vi "subGetItemInfosFromProjectFile.vi"(11 "All Files in Dir":path[](array[path])) -> (1 "Source dist":map{string, set{string}}(c390), 2 "TargetFile name":set{string}(c389), 3 "TargetFile info":T1)   [LabVIEW 2020, in "SolutionBuilder.lvlib"]
uses:
  SolutionBuilder.lvlib
  ItemInfo.ctl
  ProjectInfo.ctl
  FileInfo.ctl
  <vilib>/xml/Load XML File.vi
  <vilib>/xml/Close Reference(Node).vi
  <vilib>/xml/NI_XML.lvlib
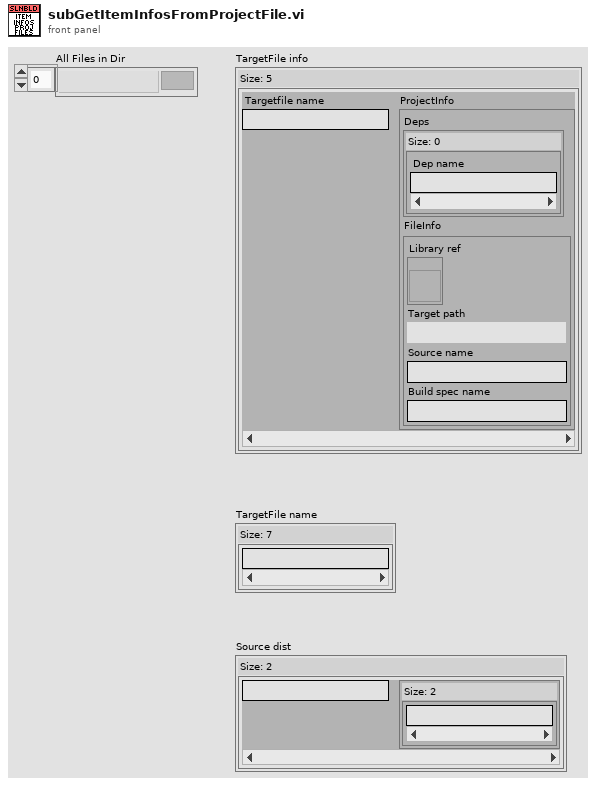
[diagram p1: front panel]
types:
  T1 = typedef "SolutionBuilder.lvlib/ItemInfo.ctl" = map{string, T2}
  T2 = typedef "SolutionBuilder.lvlib/ProjectInfo.ctl" = cluster{"Deps":set{string}, "FileInfo":T3}
  T3 = typedef "SolutionBuilder.lvlib/FileInfo.ctl" = cluster{"Library ref":refnum<vi>, "Target path":path, "Source name":string, "Build spec name":string}
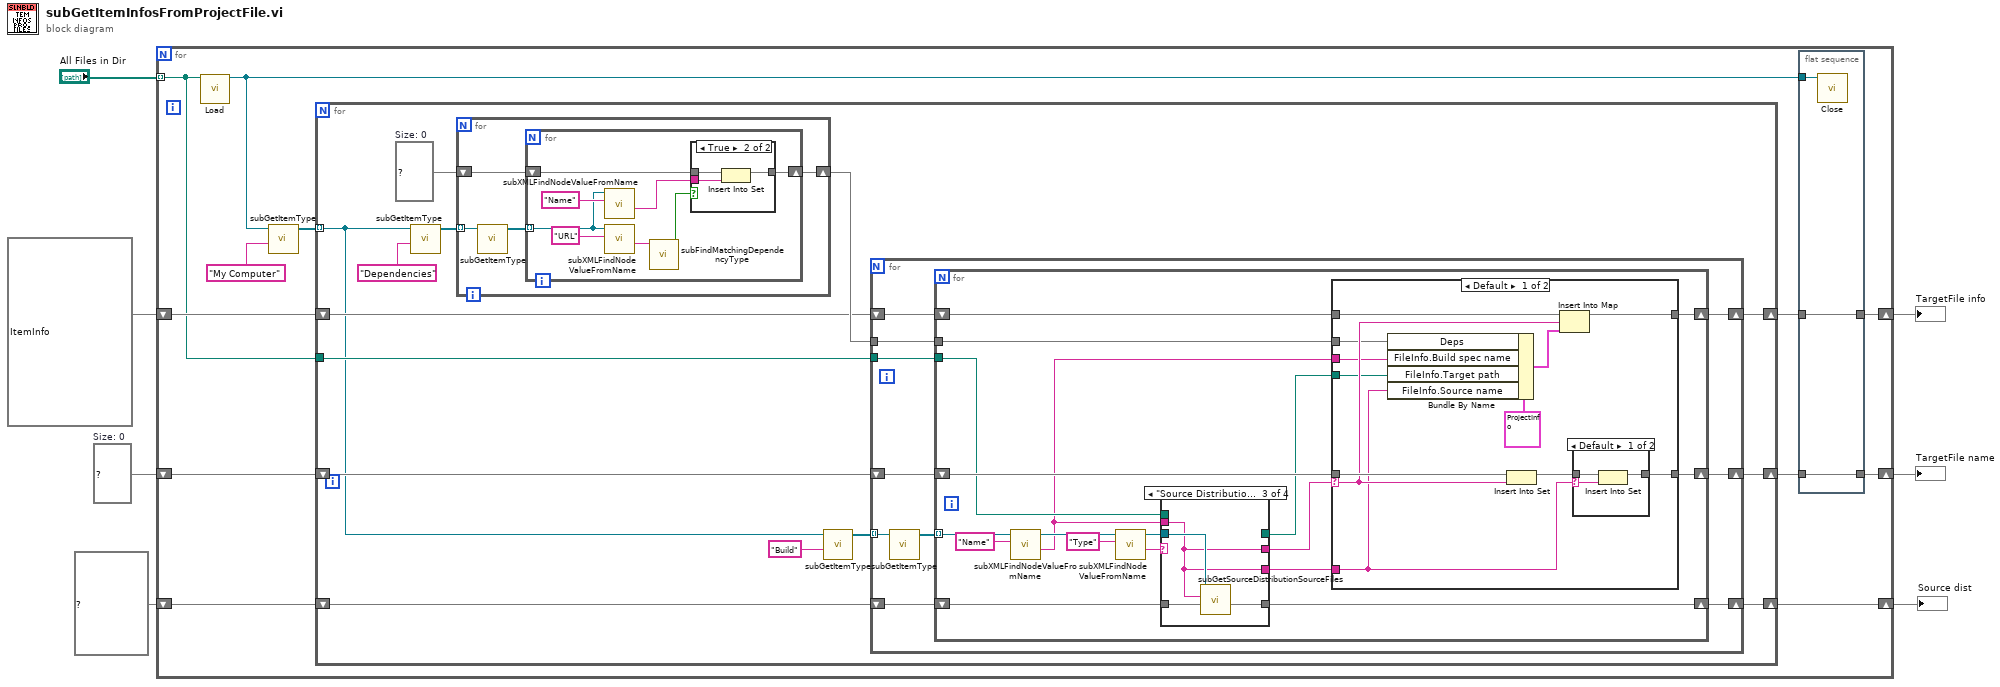
[diagram p0: block diagram]
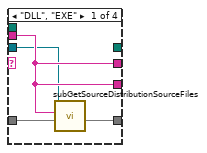
[diagram p3: hidden frame]
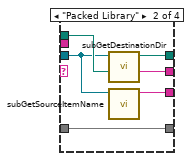
[diagram p4: hidden frame]
diagram:
  w4 = set{string} {}  # Size: 0
  n1 = for {
    tunnel: "All Files in Dir" -> [w10] mode=indexing
    shift-right: [w12] -> w5
    shift-left: w4 -> [w14]
    shift-right: [w13] -> w6
    shift-left: T1 {} ("map in") -> [w15]
    shift-right: [w9] -> w1
    shift-left: map{string, set{string}} {} ("Source dist") -> [w8]
    n2 = call-poly <vilib>:"Load.vi"("path to XML document"=w10) -> ("DOM document out"=w11:refnum<k20>)  [unwired: 12 in, 2 out]
    n3 = call "subGetItemType.vi"("Property value"="My Computer", "Refnum in"=w11) -> ("Nodes"=w18:refnum<k20>[])  [unwired: 9 in]
    n4 = for {
      tunnel: w18 -> [w27] mode=indexing
      tunnel: w10 -> [w33]
      shift-right: [w32] -> w17
      shift-left: w15 -> [w29]
      shift-right: [w31] -> w16
      shift-left: w14 -> [w28]
      shift-right: [w24] -> w9
      shift-left: w8 -> [w23]
      w36 = set{string} {}  # Size: 0
      n5 = call "subGetItemType.vi"("Property value"="Dependencies", "Refnum in"=w27) -> ("Nodes"=w25:refnum<k20>[])  [unwired: 9 in]
      n6 = for {
        tunnel: w25 -> [w40] mode=indexing
        shift-right: [w37] -> w30
        shift-left: w36 -> [w38]
        n7 = call "subGetItemType.vi"("Refnum in"=w40) -> ("Nodes"=w39:refnum<k20>[])  [unwired: 10 in]
        n8 = for {
          tunnel: w39 -> [w45] mode=indexing
          shift-right: [w41] -> w37
          shift-left: w38 -> [w44]
          n9 = call "subXMLFindNodeValueFromName.vi"("Property name"="Name", "Refnum in"=w45) -> ("Value"=w42:string)  [unwired: 7 in, 2 out]
          n10 = call "subXMLFindNodeValueFromName.vi"("Property name"="URL", "Refnum in"=w45) -> ("Value"=w47:string)  [unwired: 7 in, 2 out]
          n11 = call "subFindMatchingDependencyType.vi"("URL"=w47) -> ("Match?"=w43:bool)  [unwired: 10 in]
          n12 = case shown="True" w43 {
            tunnel: w42 -> [_ w52]
            tunnel: [w49 w51] -> w41
            tunnel: w44 -> [w49 w50]
            frame False {
            }
            frame True {
              n13 = Insert Into Set(10:w52, 11:w50) -> (3:w51:set{string})  [unwired: 1 out]
            }
          }
        }
      }
      n14 = call "subGetItemType.vi"("Property value"="Build", "Refnum in"=w27) -> ("Nodes"=w34:refnum<k20>[])  [unwired: 9 in]
      n15 = for {
        tunnel: w34 -> [w62] mode=indexing
        shift-right: [w60] -> w32
        shift-left: w29 -> [w58]
        shift-right: [w59] -> w31
        shift-left: w28 -> [w57]
        tunnel: w33 -> [w56]
        tunnel: w30 -> [w55]
        shift-right: [w54] -> w24
        shift-left: w23 -> [w53]
        n16 = call "subGetItemType.vi"("Refnum in"=w62) -> ("Nodes"=w61:refnum<k20>[])  [unwired: 10 in]
        n17 = for {
          tunnel: w61 -> [w66] mode=indexing
          shift-right: [w77] -> w60
          shift-left: w58 -> [w75]
          shift-right: [w76] -> w59
          shift-left: w57 -> [w74]
          tunnel: w56 -> [w71]
          tunnel: w55 -> [w73]
          shift-right: [w64] -> w54
          shift-left: w53 -> [w63]
          n18 = call "subXMLFindNodeValueFromName.vi"("Property name"="Name", "Refnum in"=w66) -> ("Value"=w65:string, "Refnum out"=w67:refnum<k20>)  [unwired: 7 in, 1 out]
          n19 = call "subXMLFindNodeValueFromName.vi"("Property name"="Type", "Refnum in"=w67) -> ("Value"=w79:string, "Refnum out"=w78:refnum<k20>)  [unwired: 7 in, 1 out]
          n20 = case shown="\"Source Distribution\"" w79 {
            tunnel: w78 -> [w81 w85 w94 _]
            tunnel: [w82 w89 w91 _] -> w72
            tunnel: [_ w88 _ _] -> w70
            tunnel: w71 -> [_ w90 _ _]
            tunnel: [w82 w87 w91 _] -> w69
            tunnel: w65 -> [w82 _ w91 _]
            tunnel: [w83 w86 w93 w95] -> w64
            tunnel: w63 -> [w84 w86 w92 w95]
            frame "DLL", "EXE" {
              n21 = call "subGetSourceDistributionSourceFiles.vi"("Source dist in"=w84, "Build spec name"=w82, "Refnum in"=w81) -> ("Source dist"=w83:map{string, set{string}})  [unwired: 8 in]
            }
            frame "Packed Library" {
              n22 = call "subGetDestinationDir.vi"("Project path"=w90, "Refnum in"=w85) -> ("Name"=w89:string, "Path"=w88:path)  [unwired: 8 in]
              n23 = call "subGetSourceItemName.vi"("Refnum in"=w85) -> ("source name"=w87:string)  [unwired: 10 in]
            }
            frame "Source Distribution" {
              n24 = call "subGetSourceDistributionSourceFiles.vi"("Source dist in"=w92, "Build spec name"=w91, "Refnum in"=w94) -> ("Source dist"=w93:map{string, set{string}})  [unwired: 8 in]
            }
            frame Default {
            }
          }
          n25 = case shown="Default" w72 {
            selector: w72 -> [w105 _]
            tunnel: w75 -> [w104 w113]
            tunnel: [w107 w113] -> w77
            tunnel: w74 -> [w106 w112]
            tunnel: [w102 w112] -> w76
            tunnel: w73 -> [w99 _]
            tunnel: w70 -> [w96 _]
            tunnel: w69 -> [w97 _]
            tunnel: w65 -> [w98 _]
            frame Default {
              n26 = Bundle By Name(cluster=T2 {"Deps"={}, "FileInfo"={"Library ref"=refnum, "Target path"=path "", "Source name"="", "Build spec name"=""}} ("ProjectInfo"), "Deps"=w99, "FileInfo.Build spec name"=w98, "FileInfo.Target path"=w96, "FileInfo.Source name"=w97) -> (w100:T2)
              n27 = Insert Into Set(10:w105, 11:w106) -> (3:w103:set{string})  [unwired: 1 out]
              n28 = Insert Into Map(map in=w104, key=w105, value=w100) -> (map out=w107:T1)  [unwired: 2 out]
              n29 = case shown="Default" w97 {
                selector: w97 -> [w108 _]
                tunnel: w103 -> [w110 w111]
                tunnel: [w109 w111] -> w102
                frame Default {
                  n30 = Insert Into Set(10:w108, 11:w110) -> (3:w109:set{string})  [unwired: 1 out]
                }
                frame "" {
                }
              }
            }
            frame "" {
            }
          }
        }
      }
    }
    n31 = flat-sequence {
      tunnel: w11 -> [w22]
      tunnel: w17 -> [w21]
      tunnel: w16 -> [w20]
      tunnel: [w21] -> w13
      tunnel: [w20] -> w12
      frame #0 {
        n32 = call-poly <vilib>:"Close.vi"("node"=w22) -> ()  [unwired: 8 in, 1 out]
      }
    }
  }
  "TargetFile info" <- w6
  "TargetFile name" <- w5
  "Source dist" <- w1
